vi "Station2_Data_Log.vi"(8 "error in (no error)":errorcluster, 11 "Cluster":T2) -> (0 "error out":errorcluster)   [LabVIEW 2017]
uses:
  <vilib>/addons/database/Connection.llb/Conn ObjectReference.ctl
  <vilib>/addons/database/NI_Database_API.lvlib
panel:
  out "PART 1":string
  out "PART 2":string
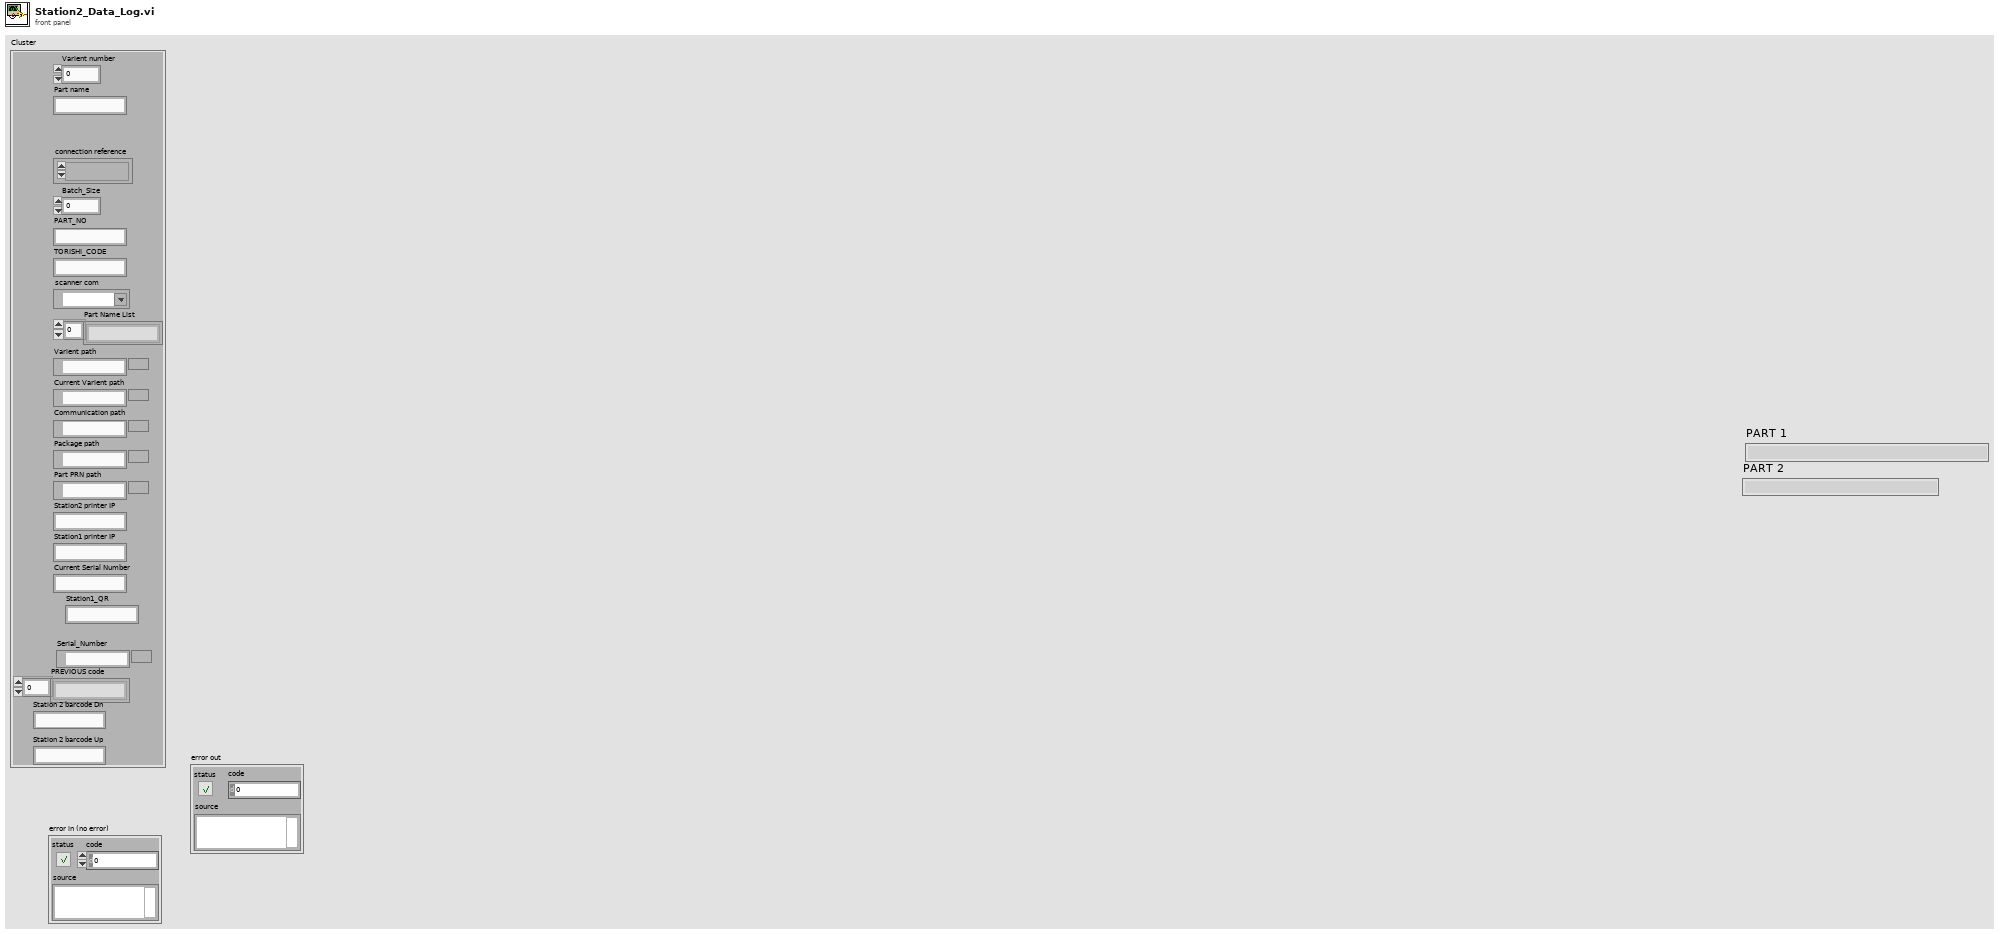
[diagram p1: front panel]
types:
  T1 = typedef "NI_Database_API.lvlib/Conn ObjectReference.ctl" = refnum<k1>
  T2 = cluster{"Varient number":u16, "Part name":string, "connection reference":T1, "Batch_Size":u16, "PART_NO":string, "TORISHI_CODE":string, "scanner com":refnum<visa-resource-name>, "Part Name List":string[], "Varient path":path, "Current Varient path":path, "Communication path":path, "Package path":path, "Part PRN path":path, "Station2 printer IP":string, "Station1 printer IP":string, "Current Serial Number":string, "Station1_QR":string, "Serial_Number":path, "PREVIOUS code":string[], "Station 2 barcode Dn":string, "Station 2 barcode Up":string}
  T3 = cluster{string, "Station 2 barcode Up":string, "Station 2 barcode Dn":string}
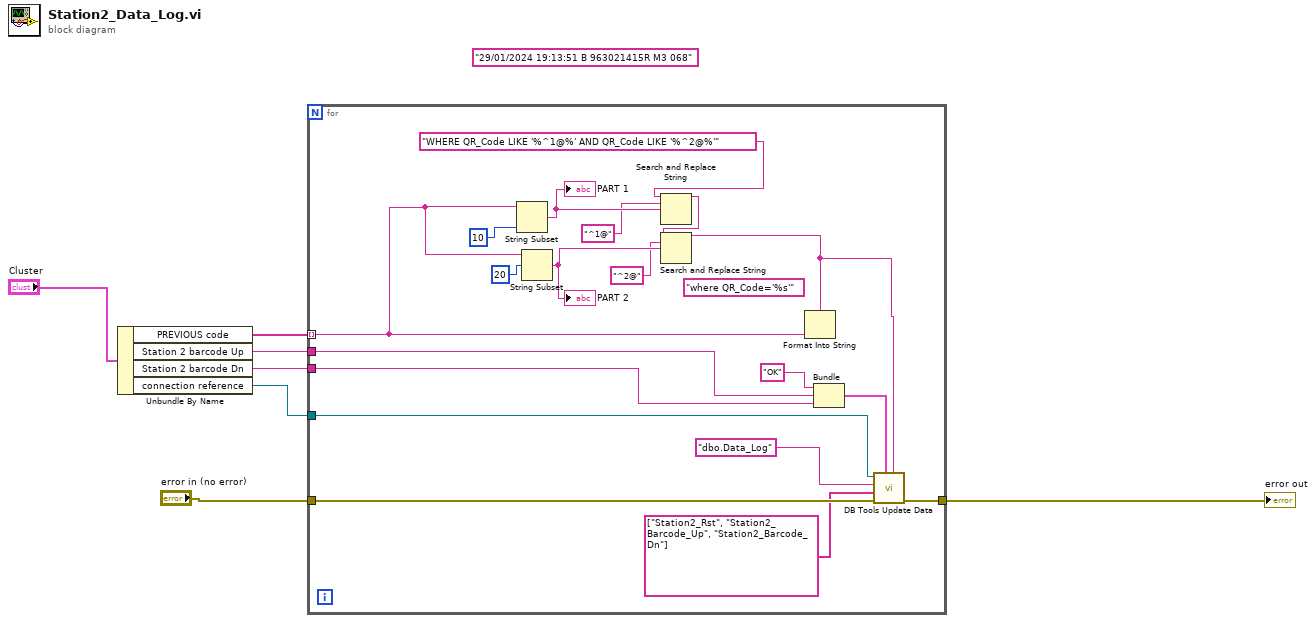
[diagram p0: block diagram]
diagram:
  (unwired) "29/01/2024 19:13:51 B 963021415R M3 068"
  n1 = Unbundle By Name("Cluster") -> ("PREVIOUS code"=w4:string[], "Station 2 barcode Up"=w3:string, "Station 2 barcode Dn"=w2:string, "connection reference"=w1:T1)
  n2 = for {
    tunnel: [w25] -> w6
    tunnel: w1 -> [w24]
    tunnel: "error in (no error)" -> [w21]
    tunnel: w4 -> [w9] mode=indexing
    tunnel: w3 -> [w20]
    tunnel: w2 -> [w19]
    (unwired) "where QR_Code='%s'" ("format string")
    n3 = String Subset(string=w9, length (rest)=10 ("offset (0)")) -> (substring=w16:string)  [unwired: 1 in]
    "PART 1" <- w16
    n4 = String Subset(string=w9, offset (0)=20) -> (substring=w17:string)  [unwired: 1 in]
    "PART 2" <- w17
    n5 = Search and Replace String(input string="WHERE QR_Code LIKE '%^1@%' AND QR_Code LIKE '%^2@%'" ("format string"), search string="^1@", replace string=w16) -> (result string=w15:string)  [unwired: 5 in, 3 out]
    n6 = Search and Replace String(input string=w15, search string="^2@", replace string=w17) -> (result string=w8:string)  [unwired: 5 in, 3 out]
    n7 = Format Into String(format string=w8, w9) -> ()  [unwired: 2 in, 2 out]
    n8 = Bundle("OK", "Station 2 barcode Up"=w20, "Station 2 barcode Dn"=w19) -> (w22:T3)  [unwired: 1 in]
    n9 = call <vilib>:"DB Tools Update Data.vi"("condition"=w8, "data"=w22, "error in (no error)"=w21, "columns"=string[] ["Station2_Rst", "Station2_Barcode_Up", "Station2_Barcode_Dn"] ("columns 2"), "table"="dbo.Data_Log", "connection reference"=w24) -> ("error out"=w25:errorcluster)  [unwired: 4 in, 1 out]
  }
  "error out" <- w6
